vi "compare readings NANOVNA.vi"() -> ()   [LabVIEW 2020]
uses:
  common/record_file_handler/VFH-VNA_File_Handler.lvlib
panel:
  out "size(s)":i32
  out "Array 3":bool[](array[boolean])
  out "Array 2":path[](array[path])
  out "S11 I":cluster{"Frequency":dbl[], "S21_Imag":dbl[]}[](graph)
  out "Magnitude":cluster{"Frequency":dbl[], "S21_Imag":dbl[]}[](graph)
  out "|Z|":cluster{"Frequency":dbl[], "S21_Imag":dbl[]}[](graph)
  out "S11 R":cluster{"Frequency":dbl[], "S21_Imag":dbl[]}[](graph)
  in  "Signal":i32
  out "Cluster":T1 {"Z''" format="%#_5p"; "Z'" format="%#_5p"; "|Z|" format="%#_5p"; "Loss" format="%#_5p"; "Deg" format="%#_5p"; "Phi" format="%#_5p"; "Mag" format="%#_5p"; "S11 I" format="%#_5p"; "S11 R" format="%#_5p"}
  out "Array":dbl[](array[numeric]) format="%#_5p"
  out "Freq":dbl format="%#_6p"
  in  "index":i32
  in  "Stop":bool
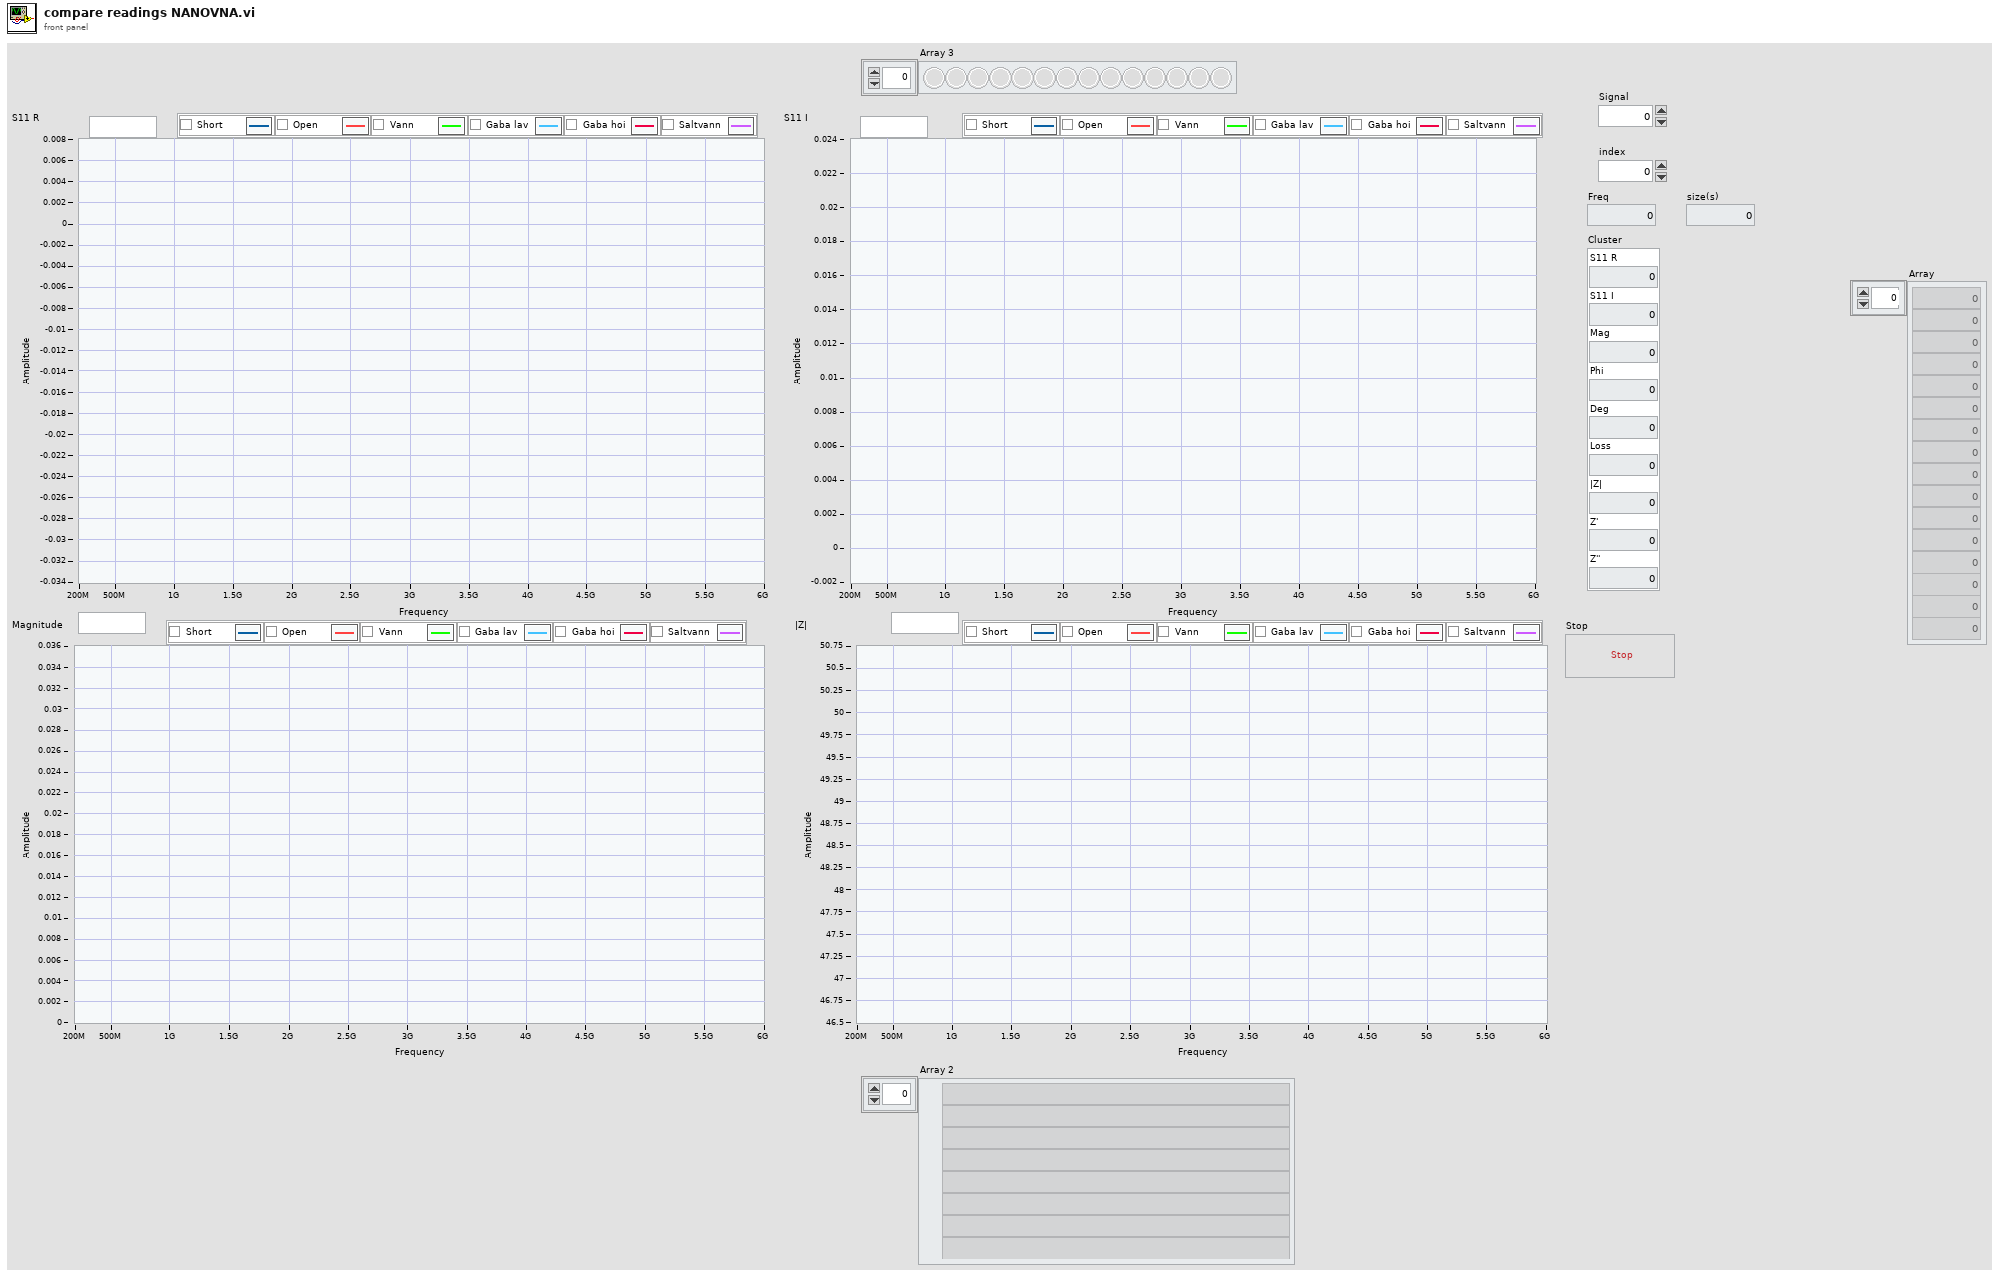
[diagram p1: front panel]
types:
  T1 = cluster{"S11 R":dbl, "S11 I":dbl, "Mag":dbl, "Phi":dbl, "Deg":dbl, "Loss":dbl, "|Z|":dbl, "Z'":dbl, "Z''":dbl}
  T2 = typedef "VFH-VNA_File_Handler.lvlib/VFH-file_cluster-NanoVNA.ctl" = cluster{"Frequency":dbl[], "S11_Real":dbl[], "S11_Imag":dbl[], "S21_Real":dbl[], "S21_Imag":dbl[], "S12_Real":dbl[], "S12_Imag":dbl[], "S22_Real":dbl[], "S22_Imag":dbl[]}
  T3 = cluster{"Loss":cluster{"Frequency":dbl[], "Array":dbl[]}, "Z Modulus":cluster{"Frequency":dbl[], "Array":dbl[]}, "Z'":cluster{"Frequency":dbl[], "Array":dbl[]}, "Z''":cluster{"Frequency":dbl[], "Array":dbl[]}}
  T4 = cluster{"S11'":cluster{"Frequency":dbl[], "S11_Real":dbl[]}, "S11''":cluster{"Frequency":dbl[], "S11_Real":dbl[]}, "Magnitude":cluster{"Frequency":dbl[], "Array":dbl[]}, "Eta":cluster{"Frequency":dbl[], "Array":dbl[]}, "Phase":cluster{"Frequency":dbl[], "Array":dbl[]}}
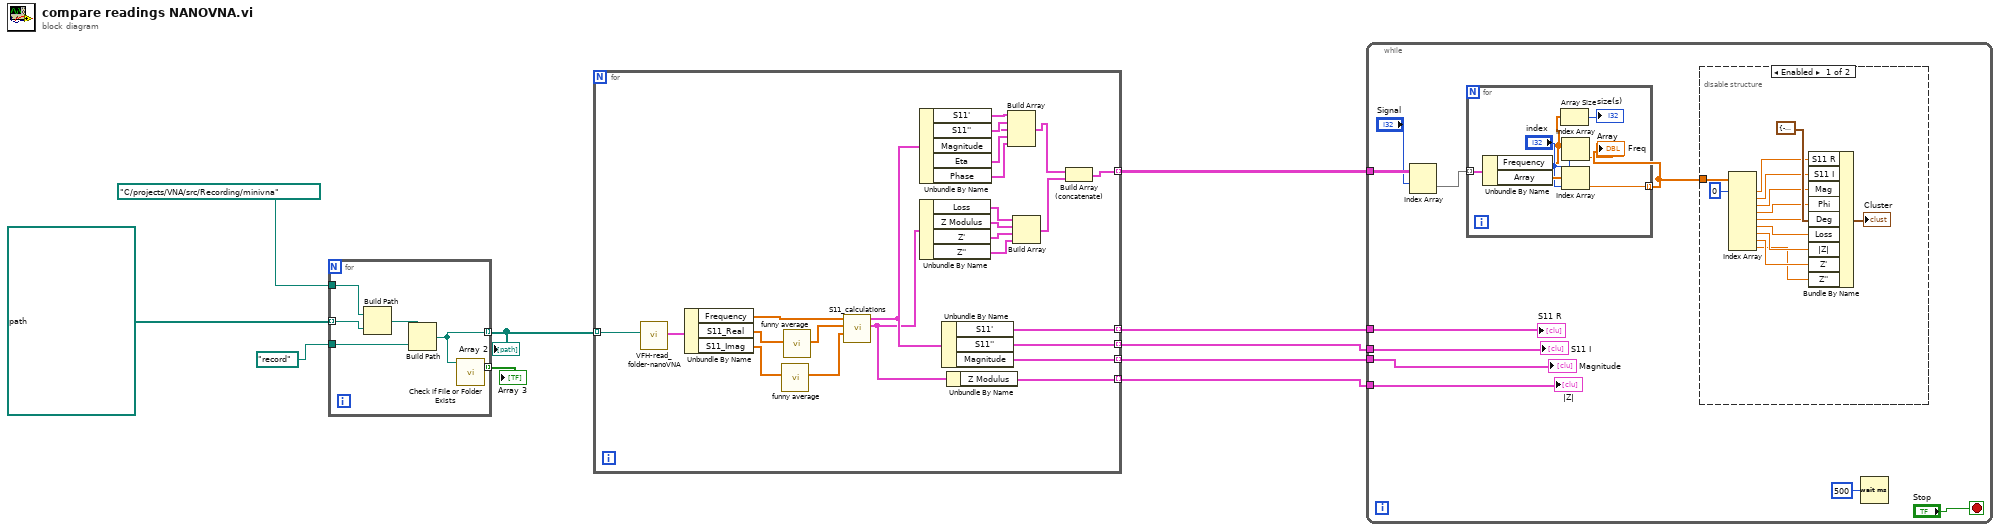
[diagram p0: block diagram]
diagram:
  n1 = for {
    tunnel: path[] [path "test-short", path "test-open", path "test-Vann", path "test-Gabalav", path "test-gabahøy", path "test-Saltvann"] ("Folder Path") -> [w15] mode=indexing
    tunnel: path "C:/projects/VNA/src/Recording/minivna" ("Folder Path") -> [w16]
    tunnel: [w12] -> w3 mode=indexing
    tunnel: [w14] -> w2 mode=indexing
    tunnel: path "record" ("name or relative path") -> [w11]
    n2 = Build Path(base path=w16, name or relative path=w15) -> (appended path=w13:path)
    n3 = Build Path(base path=w13, name or relative path=w11) -> (appended path=w12:path)
    n4 = call <vilib>:"Check if File or Folder Exists.vi"("path"=w12) -> ("file or folder exists?"=w14:bool)  [unwired: 8 in, 2 out]
  }
  "Array 2" <- w3
  "Array 3" <- w2
  n5 = for {
    tunnel: w3 -> [w27] mode=indexing
    tunnel: [w25] -> w10 mode=indexing
    tunnel: [w24] -> w9 mode=indexing
    tunnel: [w23] -> w7 mode=indexing
    tunnel: [w22] -> w8 mode=indexing
    tunnel: [w21] -> w6 mode=indexing
    n6 = call "VFH-read_folder-nanoVNA.vi"("Folder Path"=w27) -> ("avg output"=w26:T2)  [unwired: 8 in, 2 out]
    n7 = Unbundle By Name(w26) -> ("Frequency"=w41:dbl[], "S11_Real"=w20:dbl[], "S11_Imag"=w18:dbl[])
    n8 = call "funny average.vi"("in"=w18) -> ("Out"=w17:dbl[])  [unwired: 10 in]
    n9 = call "funny average.vi"("in"=w20) -> ("Out"=w19:dbl[])  [unwired: 10 in]
    n10 = call "S11_calculations.vi"("S11_Imag"=w17, "S11_Real"=w19, "Frequency"=w41) -> ("Calc"=w28:T3, "Raw"=w29:T4)  [unwired: 6 in, 1 out]
    n11 = Unbundle By Name(w29) -> ("S11'"=w40:cluster{"Frequency":dbl[], "S11_Real":dbl[]}, "S11''"=w39:cluster{"Frequency":dbl[], "S11_Real":dbl[]}, "Magnitude"=w38:cluster{"Frequency":dbl[], "Array":dbl[]}, "Eta"=w37:cluster{"Frequency":dbl[], "Array":dbl[]}, "Phase"=w36:cluster{"Frequency":dbl[], "Array":dbl[]})
    n12 = Unbundle By Name(w28) -> ("Loss"=w35:cluster{"Frequency":dbl[], "Array":dbl[]}, "Z Modulus"=w34:cluster{"Frequency":dbl[], "Array":dbl[]}, "Z'"=w33:cluster{"Frequency":dbl[], "Array":dbl[]}, "Z''"=w32:cluster{"Frequency":dbl[], "Array":dbl[]})
    n13 = Unbundle By Name(w29) -> ("S11'"=w25:cluster{"Frequency":dbl[], "S11_Real":dbl[]}, "S11''"=w24:cluster{"Frequency":dbl[], "S11_Real":dbl[]}, "Magnitude"=w23:cluster{"Frequency":dbl[], "Array":dbl[]})
    n14 = Unbundle By Name(w28) -> ("Z Modulus"=w22:cluster{"Frequency":dbl[], "Array":dbl[]})
    n15 = Build Array(w40, w39, w38, w37, w36) -> (w30:cluster{"Frequency":dbl[], "Array":dbl[]}[])
    n16 = Build Array(w35, w34, w33, w32) -> (w31:cluster{"Frequency":dbl[], "Array":dbl[]}[])
    n17 = Build Array (concatenate)(w30, w31) -> (w21:cluster{"Frequency":dbl[], "Array":dbl[]}[])
  }
  n18 = while {
    tunnel: w10 -> [w51]
    tunnel: w9 -> [w50]
    tunnel: w8 -> [w49]
    tunnel: w7 -> [w48]
    tunnel: w6 -> [w46]
    stop <- "Stop" stop-if-true
    n19 = Index Array(array=w46, index (row)="Signal") -> (element=w45:cluster{"Frequency":dbl[], "Array":dbl[]}[])  [unwired: 1 in]
    n20 = for {
      tunnel: w45 -> [w58] mode=indexing
      tunnel: [w54] -> w47 mode=indexing
      n21 = Unbundle By Name(w58) -> ("Frequency"=w53:dbl[], "Array"=w57:dbl[])
      n22 = Array Size(array=w53) -> (size(s)=→"size(s)":i32)
      n23 = Index Array(array=w53, index="index") -> (element=→"Freq":dbl)
      n24 = Index Array(array=w57, index="index") -> (element=w54:dbl)
    }
    "Array" <- w47
    n25 = disable-structure shown="Enabled" {
      disable-tunnel: w47 -> [w71 _]
      frame Enabled {
        n26 = Index Array(array=w71, index #1=0 ("index (row)")) -> (element #1=w68:dbl, element #2=w67:dbl, element #3=w66:dbl, element #4=w65:dbl, element #5=w64:dbl, element #6=w63:dbl, element #7=w62:dbl, element #8=w61:dbl, element #9=w60:dbl)  [unwired: 8 in]
        n27 = Bundle By Name(cluster=T1 {"S11 R"=-0.13079270605384616, "S11 I"=-0.13079270605384616, "Mag"=-0.13079270605384616, "Phi"=-0.13079270605384616, "Deg"=-0.13079270605384616, "Loss"=-0.13079270605384616, "|Z|"=-0.13079270605384616, "Z'"=-0.13079270605384616, "Z''"=-0.13079270605384616} ("Cluster"), "S11 R"=w68, "S11 I"=w67, "Mag"=w66, "Phi"=w65, "Deg"=w64, "Loss"=w63, "|Z|"=w62, "Z'"=w61, "Z''"=w60) -> (→"Cluster":T1)
      }
      frame Disabled {
      }
    }
    n28 = Wait (ms)(milliseconds to wait=u32 500) -> ()  [unwired: 1 out]
    "Magnitude" <- w48
    "S11 R" <- w51
    "|Z|" <- w49
    "S11 I" <- w50
  }
